vi "Is Connected.vi"(8 "error in":errorcluster, 11 "NetStream in":refnum<class "NetStream.lvclass">) -> (0 "error out":errorcluster, 2 "Connected?":bool, 3 "NetStream out":refnum<class "NetStream.lvclass">)   [LabVIEW 2020, in "hse-network.lvlib" / "NetStream.lvclass"]
doc: "____\nHAMPEL SOFTWARE ENGINEERING v3.8.0 (2023-12-18 14:41)"
uses:
  NetStream.lvclass
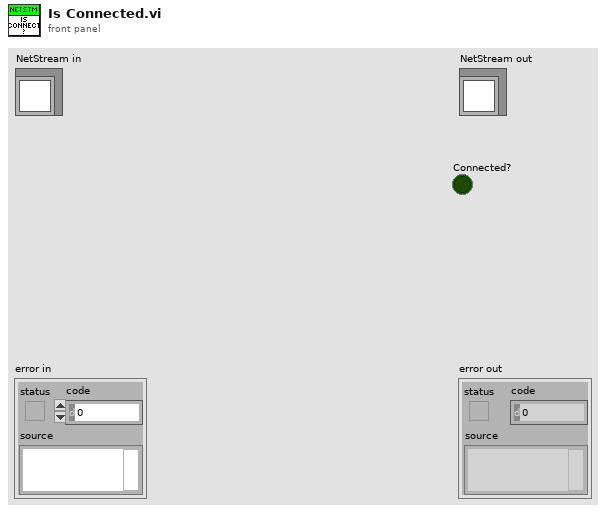
[diagram p1: front panel]
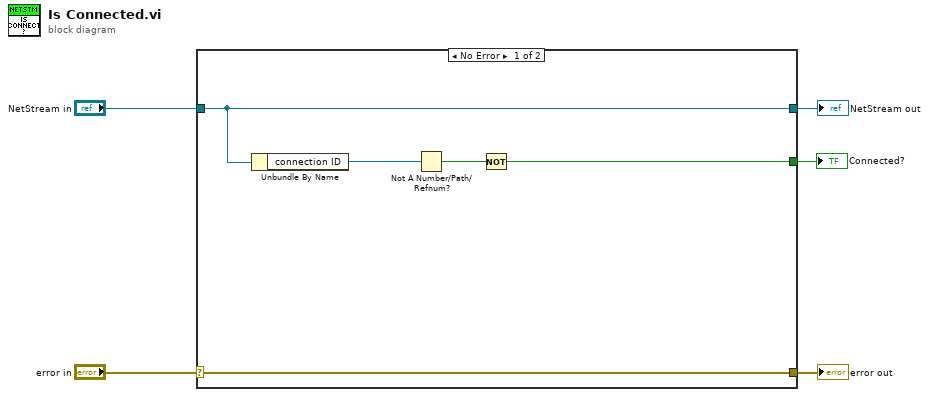
[diagram p0: block diagram]
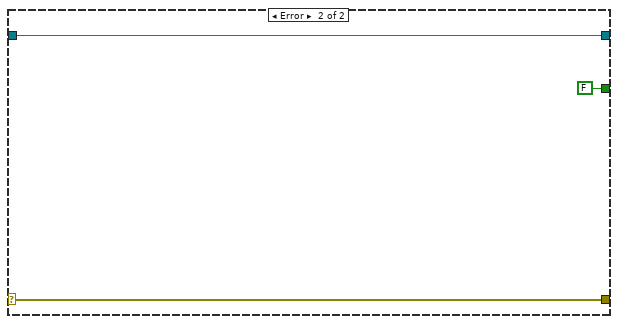
[diagram p2: hidden frame]
diagram:
  n1 = case shown="No Error" "error in" {
    selector: "error in" -> [w10 w13]
    tunnel: [w10 w13] -> w4
    tunnel: [w9 w12] -> w2
    tunnel: "NetStream in" -> [w9 w12]
    tunnel: [w6 FALSE] -> w1
    frame No Error {
      n2 = Unbundle By Name(w9) -> ("connection ID"=w8:refnum<k5>)
      n3 = Not A Number/Path/Refnum?(number/path/refnum=w8) -> (NaN/Path/Refnum?=w7:bool)
      n4 = Not(x=w7) -> (.not. x?=w6:bool)
    }
    frame Error {
    }
  }
  "error out" <- w4
  "NetStream out" <- w2
  "Connected?" <- w1
